vi "Main.vi"   [LabVIEW 2020, in "Display As.lvlib"]
uses:
  Display As.lvlib
  DA Child A/DA Child A.lvclass
  C:/dev/LabVIEW/lv-oopanel/Examples/Display As/DA Parent/DA Parent.lvclass
  DA Child B/DA Child B.lvclass
  DA Parent/DA Parent.lvclass
  C:/dev/LabVIEW/lv-oopanel/OOPanel/ArrayPanel/ArrayPanel.lvclass
  OOPanel/ArrayManager/ArrayManager.lvclass
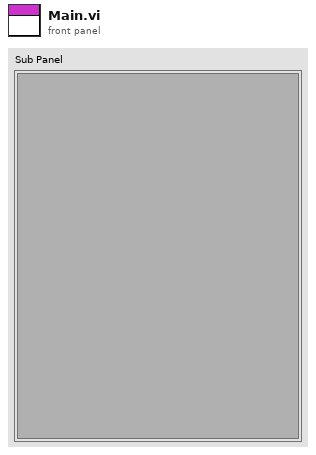
[diagram p1: front panel]
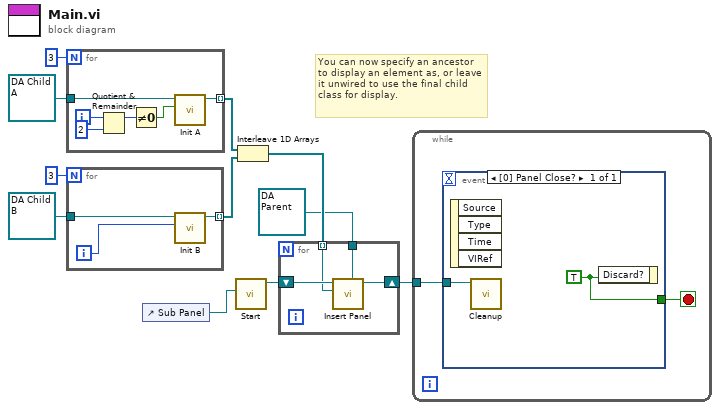
[diagram p0: block diagram]
diagram:
  # "You can now specify an ancestor to display an element as, or leave it unwired to use the final child class for display."
  n1 = for {
    N: 3 -> [_]
    tunnel: refnum<class "DA Child A.lvclass"> refnum ("Display As.lvlib:DA Child A.lvclass") -> [w14]
    tunnel: [w12] -> w5 mode=indexing
    i -> [w17]
    n2 = Quotient & Remainder(x=w17, y=2) -> (x-y*floor(x/y)=w15:i32)  [unwired: 1 out]
    n3 = Not Equal To 0?(x=w15) -> (x != 0?=w13:bool)
    n4 = call "Init A.vi"("Boolean"=w13, "DA Child A in"=w14) -> ("DA Child A out"=w12:refnum<class "DA Child A.lvclass">)  [unwired: 8 in, 1 out]
  }
  n5 = for {
    N: 3 -> [_]
    tunnel: refnum<class "DA Child B.lvclass"> refnum ("Display As.lvlib:DA Child B.lvclass") -> [w20]
    tunnel: [w18] -> w4 mode=indexing
    i -> [w19]
    n6 = call "Init B.vi"("Numeric"=w19, "DA Child B in"=w20) -> ("DA Child B out"=w18:refnum<class "DA Child B.lvclass">)  [unwired: 8 in, 1 out]
  }
  n7 = control-ref of="Sub Panel"() -> (w11:refnum<vi>)
  n8 = call "Start.vi"("Container"=w11) -> ("ArrayManager out"=w10:refnum<class "ArrayManager.lvclass">)  [unwired: 9 in, 1 out]
  n9 = Interleave 1D Arrays(w5, w4) -> (w3:refnum<class "DA Parent.lvclass">[])
  n10 = for {
    shift-right: [w22] -> w2
    shift-left: w10 -> [w24]
    tunnel: w3 -> [w23] mode=indexing
    tunnel: refnum<class "DA Parent.lvclass"> refnum ("Display As.lvlib:DA Parent.lvclass") -> [w21]
    n11 = call "Insert Panel.vi"("Display Type"=w21, "Panel/Type"=w23, "PanelArray in"=w24) -> ("PanelArray out"=w22:refnum<class "ArrayManager.lvclass">)  [unwired: 6 in, 2 out]
  }
  n12 = while {
    tunnel: w2 -> [w26]
    stop <- w25 stop-if-true
    n13 = event shown="[0] Panel Close?" {
      selector: _ -> [_]
      dyn-events: _ -> [_]
      timeout: _ -> [_]
      tunnel: w26 -> [w27]
      tunnel: [w28] -> w25
      event Panel Close? {
        w28 = TRUE
        n14 = event-data() -> ()  [unwired: 1 in, 4 out]
        n15 = call "Cleanup.vi"("PanelArray in"=w27) -> ()  [unwired: 8 in, 3 out]
        n16 = event-data("Discard?"=w28) -> ()  [unwired: 1 in, 1 out]
      }
    }
  }
